vi "write_test_section_data.vi"(0 "dequeued data":T2={"Vapor Flow rate [g/s]"=0.0, "Liquid Flow rate [g/s]"=0.0, "Pressure/Temperature/Mixture Properties"={"Line Densities\n[g/cm^3]"={"Vapor Line"=-0.5709072724525495, "Liquid Line"=-0.47632842474153186}, "Mixture Properties"={"Enthalpy"=750619.9078232183, "Quality [-]"=0.5582470994443012}, "Component PTs"={"Liquid Tank P"=75343.41840909192, "Liquid Tank T"=30.52089213992321, "Liquid Tank Sat P"=181672.1439612281, "Liquid Tank Sat T"=6.822433775844459, "Separator P"=74401.45263172078, "Separator T"=37.19266445537589, "Separator Sat P"=233689.11712149414, "Separator Sat T"=6.478325372998782, "Liquid Inlet P"=82835.85841564724, "Liquid Inlet T"=193.56636718774698, "Liquid Inlet Sat P"=85427705.90320142, "Liquid Inlet Sat T"=9.415449685318322, "Vapor Tank P"=97469.18687679394, "Vapor Tank T"=6.224572479514193, "Vapor Tank Sat P"=72622.70102329315, "Vapor Tank Sat T"=13.864813139764351, "Vapor Inlet P"=182393.24586324493, "Vapor Inlet T"=24.91728208875432, "Vapor Inlet Sat P"=147043.33437190636, "Vapor Inlet Sat T"=31.003861452545706, "Test Section P"=nan, "Test Section T"=nan, "Test Section Sat P"=nan, "Test Section Sat T"=nan, "Upper Dev Section P"=14144.091653823736, "Upper Dev Section T"=549.9665015569866, "Upper Dev Section Sat P"=59290643216604.28, "Upper Dev Section Sat T"=-38.9295482785942, "Lower Dev Section P"=11233.297245789605, "Lower Dev Section T"=-2772.217721215085, "Lower Dev Section Sat P"=2.101296208665166e-41, "Lower Dev Section Sat T"=-45.23166544765655}, "Ambient Pressure [Pa]"=34261.54460917978, "Mixing Tee"={"Mixing Tee dP"=0.0, "PG inlet-Mixing Tee Abs Pressure"=0.0, "PG inlet-Mixing Tee Temperature"=0.0}}, "Seconds Since \nSession Start"=0.0}, 1 "Loop Data Labels":string[](array[string])=["Vap Mass Flow", "Liq Mass Flow", "DP", "Liq Tank P", "LiqTank T", "Sep P", "SepT", "Liq In P", "Liq In T", "Vap Tank P", "Vap Tank T", "Dev Section P", "Dev Section T", "Up TS P", "Up TS T", "Low TS P", "Low TS T", "Cond Top T", "Evap Top T", "Cond Bot T", "Evap Bot T", "Win 3-4 P", "Top Heat T", "Bot Heat T"], 2 "Loop Data Index":dbl, 3 "Loop Data Prefix":string, 4 "Loop Data Folder":path) -> ()   [LabVIEW 2017]
uses:
  <vilib>/Utility/file.llb/Write Delimited Spreadsheet (DBL).vi
  pressure_temp_mixture.ctl
panel:
  # "Saturation\nPressure [Pa]"
  # "Saturation\nTemperature [C]"
  # "Pressure [Pa]"
  # "Temperature [C]"
  # "Liquid Tank"
  # "Separator"
  # "Liquid Inlet"
  # "Vapor Tank"
  # "Vapor Inlet"
  # "Test Section"
  # "Upper Dev Section"
  # "Lower Dev Section"
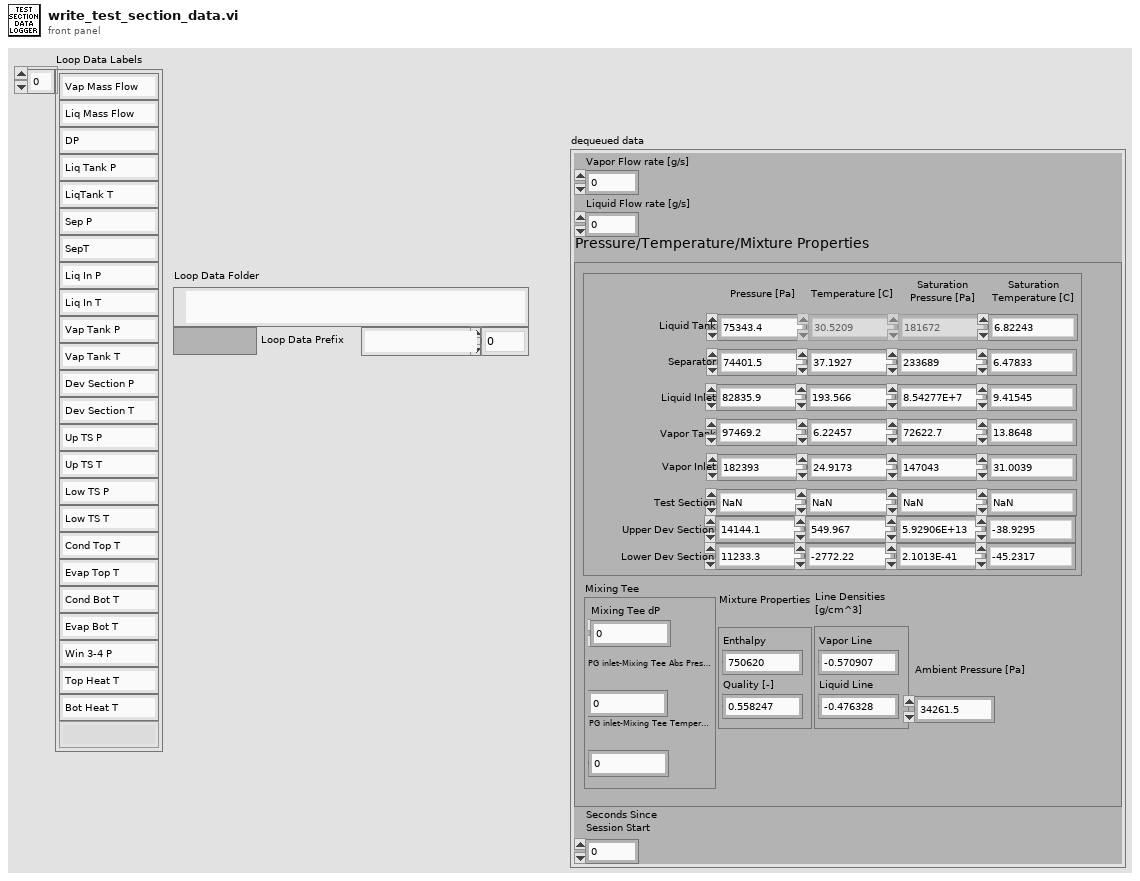
[diagram p1: front panel]
types:
  T1 = typedef "pressure_temp_mixture.ctl" = cluster{"Line Densities\n[g/cm^3]":cluster{"Vapor Line":dbl, "Liquid Line":dbl}, "Mixture Properties":cluster{"Enthalpy":dbl, "Quality [-]":dbl}, "Component PTs":cluster{"Liquid Tank P":dbl, "Liquid Tank T":dbl, "Liquid Tank Sat P":dbl, "Liquid Tank Sat T":dbl, "Separator P":dbl, "Separator T":dbl, "Separator Sat P":dbl, "Separator Sat T":dbl, "Liquid Inlet P":dbl, "Liquid Inlet T":dbl, "Liquid Inlet Sat P":dbl, "Liquid Inlet Sat T":dbl, "Vapor Tank P":dbl, "Vapor Tank T":dbl, "Vapor Tank Sat P":dbl, "Vapor Tank Sat T":dbl, "Vapor Inlet P":dbl, "Vapor Inlet T":dbl, "Vapor Inlet Sat P":dbl, "Vapor Inlet Sat T":dbl, "Test Section P":dbl, "Test Section T":dbl, "Test Section Sat P":dbl, "Test Section Sat T":dbl, "Upper Dev Section P":dbl, "Upper Dev Section T":dbl, "Upper Dev Section Sat P":dbl, "Upper Dev Section Sat T":dbl, "Lower Dev Section P":dbl, "Lower Dev Section T":dbl, "Lower Dev Section Sat P":dbl, "Lower Dev Section Sat T":dbl}, "Ambient Pressure [Pa]":dbl, "Mixing Tee":cluster{"Mixing Tee dP":dbl, "PG inlet-Mixing Tee Abs Pressure":dbl, "PG inlet-Mixing Tee Temperature":dbl}}
  T2 = cluster{"Vapor Flow rate [g/s]":dbl, "Liquid Flow rate [g/s]":dbl, "Pressure/Temperature/Mixture Properties":T1, "Seconds Since \nSession Start":dbl}
  T3 = cluster{"Liquid Tank P":dbl, "Liquid Tank T":dbl, "Liquid Tank Sat P":dbl, "Liquid Tank Sat T":dbl, "Separator P":dbl, "Separator T":dbl, "Separator Sat P":dbl, "Separator Sat T":dbl, "Liquid Inlet P":dbl, "Liquid Inlet T":dbl, "Liquid Inlet Sat P":dbl, "Liquid Inlet Sat T":dbl, "Vapor Tank P":dbl, "Vapor Tank T":dbl, "Vapor Tank Sat P":dbl, "Vapor Tank Sat T":dbl, "Vapor Inlet P":dbl, "Vapor Inlet T":dbl, "Vapor Inlet Sat P":dbl, "Vapor Inlet Sat T":dbl, "Test Section P":dbl, "Test Section T":dbl, "Test Section Sat P":dbl, "Test Section Sat T":dbl, "Upper Dev Section P":dbl, "Upper Dev Section T":dbl, "Upper Dev Section Sat P":dbl, "Upper Dev Section Sat T":dbl, "Lower Dev Section P":dbl, "Lower Dev Section T":dbl, "Lower Dev Section Sat P":dbl, "Lower Dev Section Sat T":dbl}
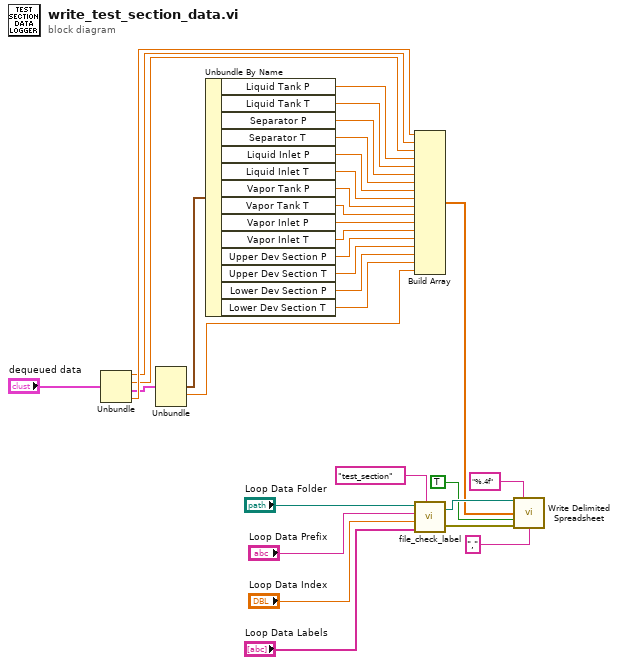
[diagram p0: block diagram]
diagram:
  n1 = Unbundle("dequeued data") -> ("Vapor Flow rate [g/s]"=w4:dbl, "Liquid Flow rate [g/s]"=w5:dbl, "Pressure/Temperature/Mixture Properties"=w6:T1, "Seconds Since \nSession Start"=w28:dbl)
  n2 = Unbundle(w6) -> ("Component PTs"=w7:T3, "Ambient Pressure [Pa]"=w1:dbl)  [unwired: 3 out]
  n3 = Unbundle By Name(w7) -> ("Liquid Tank P"=w8:dbl, "Liquid Tank T"=w9:dbl, "Separator P"=w10:dbl, "Separator T"=w11:dbl, "Liquid Inlet P"=w12:dbl, "Liquid Inlet T"=w13:dbl, "Vapor Tank P"=w14:dbl, "Vapor Tank T"=w15:dbl, "Vapor Inlet P"=w16:dbl, "Vapor Inlet T"=w17:dbl, "Upper Dev Section P"=w18:dbl, "Upper Dev Section T"=w19:dbl, "Lower Dev Section P"=w20:dbl, "Lower Dev Section T"=w21:dbl)
  n4 = Build Array(w28, w4, w5, w8, w9, w10, w11, w12, w13, w14, w15, w16, w17, w18, w19, w20, w21, w1) -> (w22:dbl[])
  n5 = call "file_check_label.vi"("base path"="Loop Data Folder", "prefix"="Loop Data Prefix", "index"="Loop Data Index", "Loop Data Labels"="Loop Data Labels", "task name"="test_section") -> ("dup path"=w26:path, "error out"=w27:errorcluster)
  n6 = call-poly <vilib>:"Write Delimited Spreadsheet.vi"("file path (dialog if empty)"=w26, "format (%.3f)"="%.4f", "1D data"=w22, "append to file? (new file:F)"=TRUE ("append to file? (F)"), "error in (no error)"=w27, "delimiter (\\t)"="," ("delimiter (\\t)")) -> ()  [unwired: 8 in, 2 out]
